vi "ProEM.vi"() -> ()   [LabVIEW 2012]
uses:
  <vilib>/Utility/error.llb/DialogType.ctl
  <vilib>/Platform/TimedLoop/XDataNode/timing_clust.ctl
  <vilib>/Platform/TimedLoop/XDataNode/nitl_modes.ctl
  <vilib>/Platform/TimedLoop/XDataNode/wakeup.ctl
  SITK/Documents/SIToolkit/LabVIEW/Examples2012_4_1_0_4/Open-Close/CamHandle.vi
  <vilib>/platform/TimedLoop/XDataNode/XDataNode.xnode
  <vilib>/Platform/TimedLoop/XDataNode/XDNodeRunTimeDep.lvlib
panel:
  in  "Tab Control":enum32{"Control", "Advanced"}(tab)
  in  "?":u16(ring) items=["Debug", "Bulb Trigger", "Free Run"]
  out "Image Monitor":u16[][](graph)
  in  "Number of Accumulations":u32=1
  in  "Number of Images":u32=1
  in  "Time Between Shots":dbl
  in  "Acquire / Focus Flag":u32(ring)=2 items=["Synchronous Focus Mode"=1, "Synchronous NFrame Mode"=2, "Asynchronous Mode"=3, "Sequence Mode"=4]
  in  "Errors":errorcluster
  in  "ADC Gain":i32=-1 min=-1 step=1
  in  "ADC Speed":i32=-1 min=-3 step=1
  in  "Exposure (sec)":dbl format="%.3f"
  in  "Timing Mode":u32(ring)=4 items=["Free Run"=1, "Trigger First"=2, "Strobe"=3, "Bulb"=4, "Variable"=5, "Flash"=6]
  in  "Trigger Edge":u32(ring)=1 items=["Rising"=1, "Falling"=2]
  in  "stop":bool
  in  "Camera Handle 2":u32
  in  "File and Display Name 2":string
  in  "error in (no error) 2":errorcluster
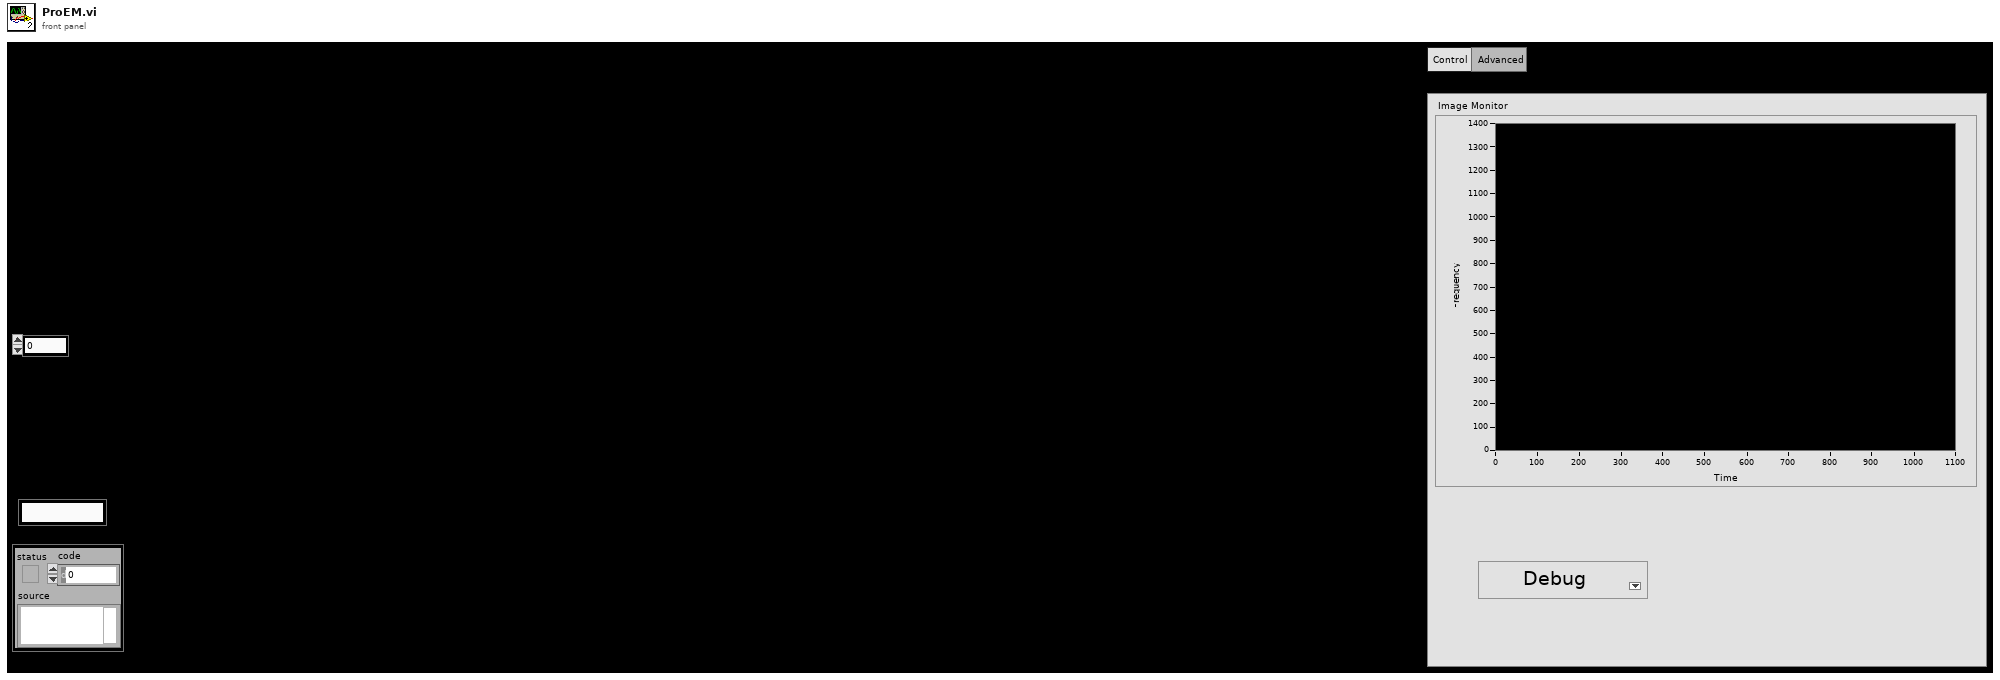
[diagram p1: front panel]
types:
  T1 = typedef "XDNodeRunTimeDep.lvlib/timing_clust.ctl" = cluster{"Expected End [f-1]":u64, "Actual End [f-1]":u64, "Finished Late? [f-1]":bool, "Expected End [i-1]":u64, "Actual End [i-1]":u64, "Finished Late? [i-1]":bool, "Expected Start [i]":u64, "Actual Start [i]":u64, "Expected Start [f]":u64, "Actual Start [f]":u64, "Source Name":string, "Structure Name":string, "Period":i64, "Deadline":i64, "Offset":i64, "Start":i64, "Priority":i32, "Timeout":i32, "Mode":T2, "Wakeup Reason":T3, "Error":errorcluster, "Source Type":string, "Secondary Source Type":string, "Global End Time":u64, "Global Start Time":u64, "Frame Duration":u64, "Iteration Duration":u64, "Assigned CPU":i32, "I/O Scan Engine Mode":u32}
  T2 = typedef "XDNodeRunTimeDep.lvlib/nitl_modes.ctl" = enum32{"No Change", "Process missed periods, maintain original phase", "Discard missed periods, maintain original phase", "Process missed periods, ignore original phase", "Discard missed periods, ignore original phase"}
  T3 = typedef "XDNodeRunTimeDep.lvlib/wakeup.ctl" = enum32{"Normal", "Aborted", "Asynchronous wakeup", "Timing source error", "Timed loop error", "Timeout"}
  T4 = typedef "DialogType.ctl" = u16
  T5 = cluster{"Camera Handle":u32, "File Handle":u32, "Display Handle":u32, "Image Handle":u32}
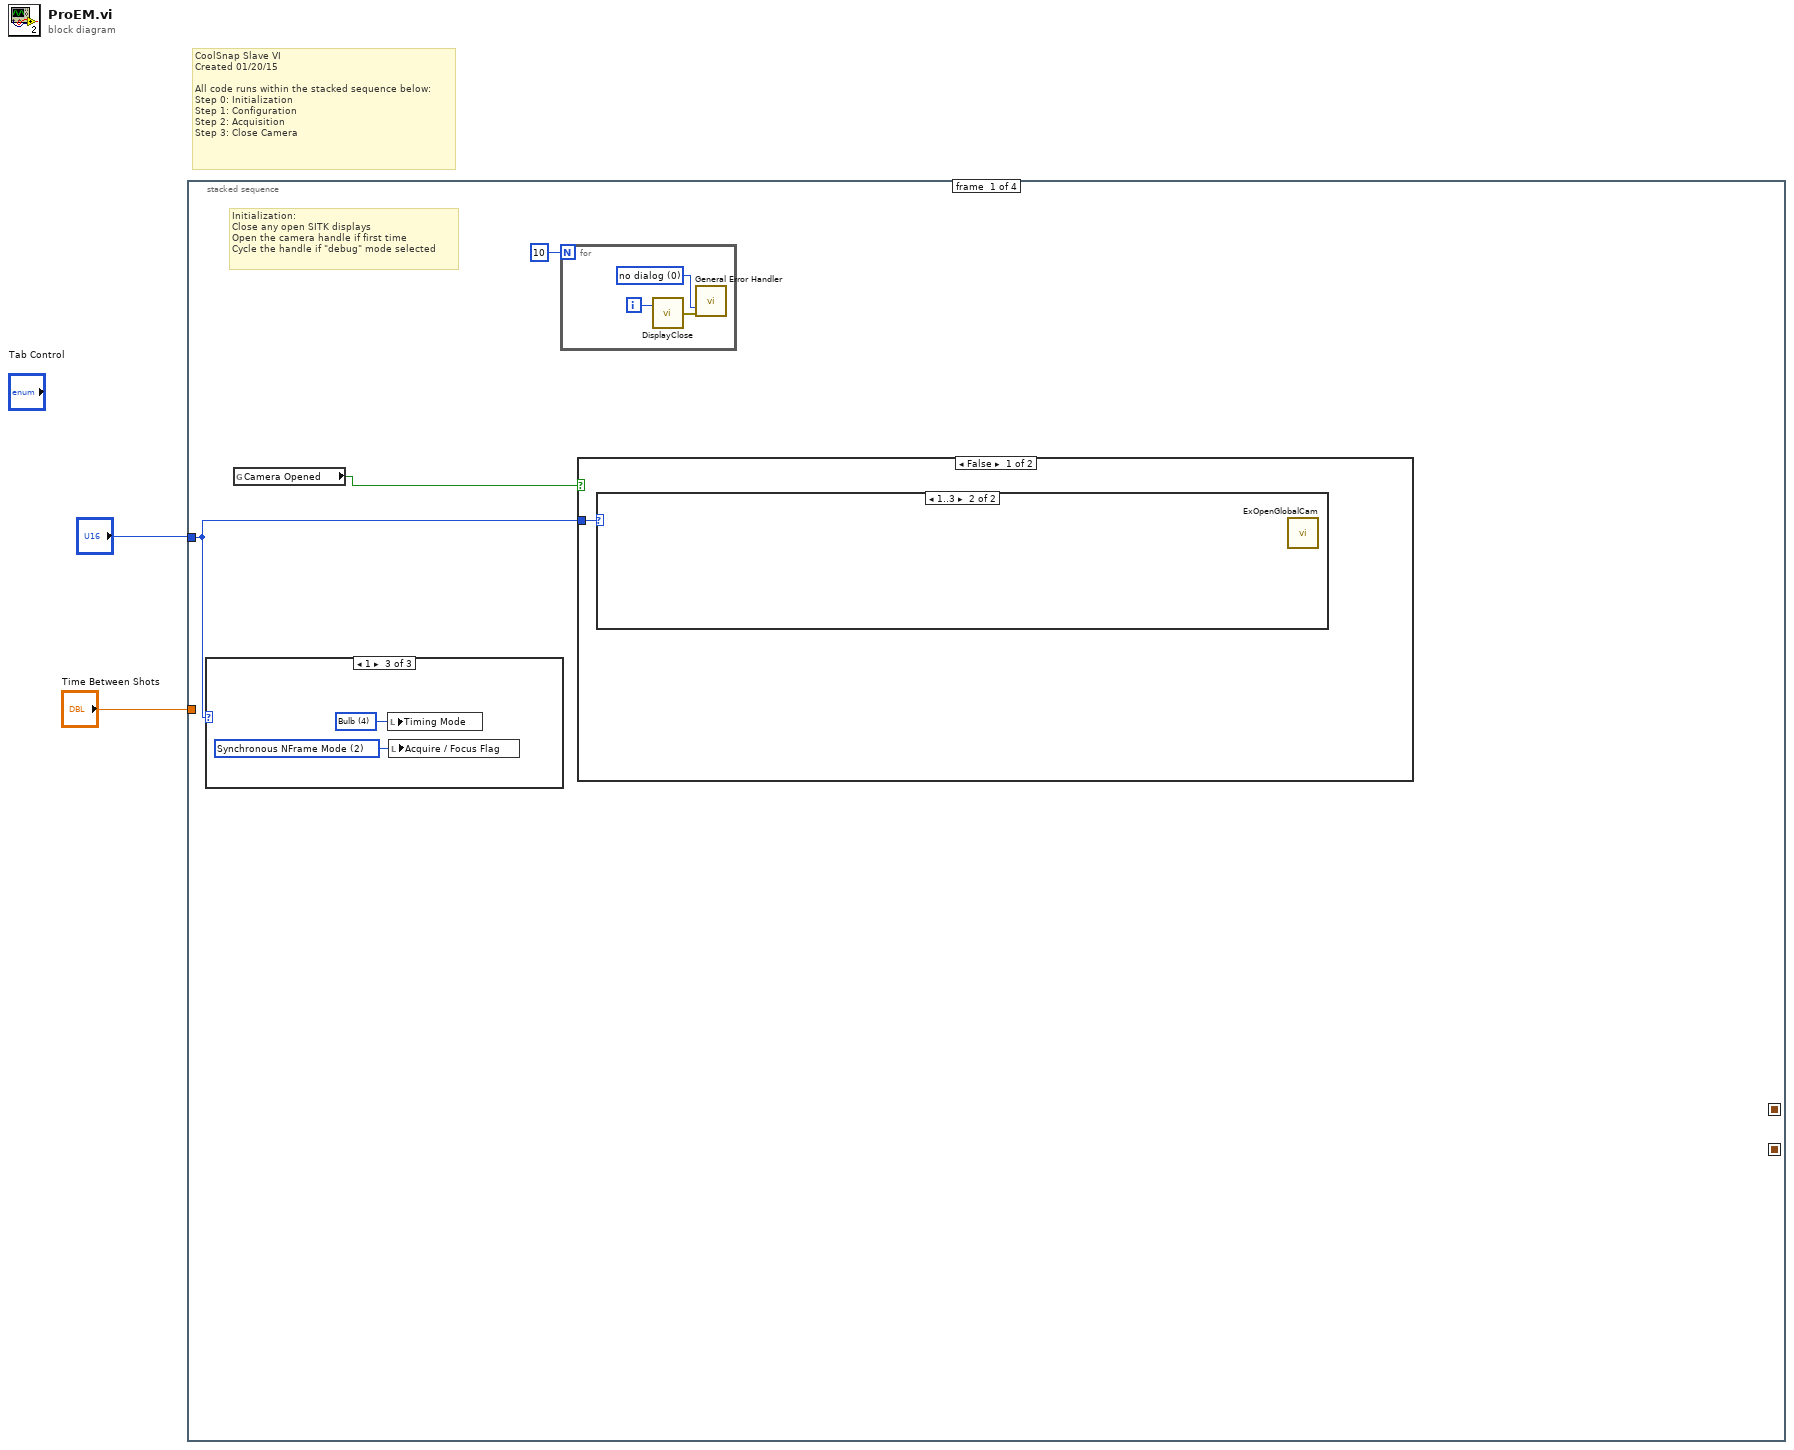
[diagram p0: block diagram]
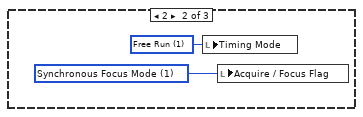
[diagram p3: hidden frame]
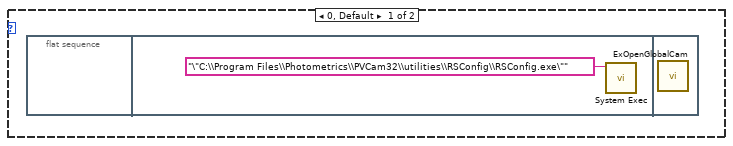
[diagram p4: hidden frame]
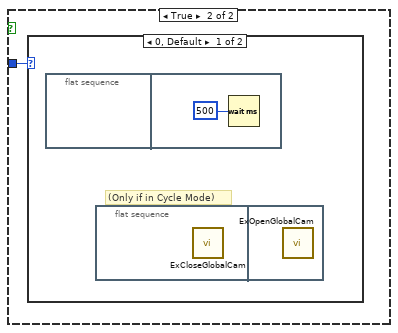
[diagram p5: hidden frame]
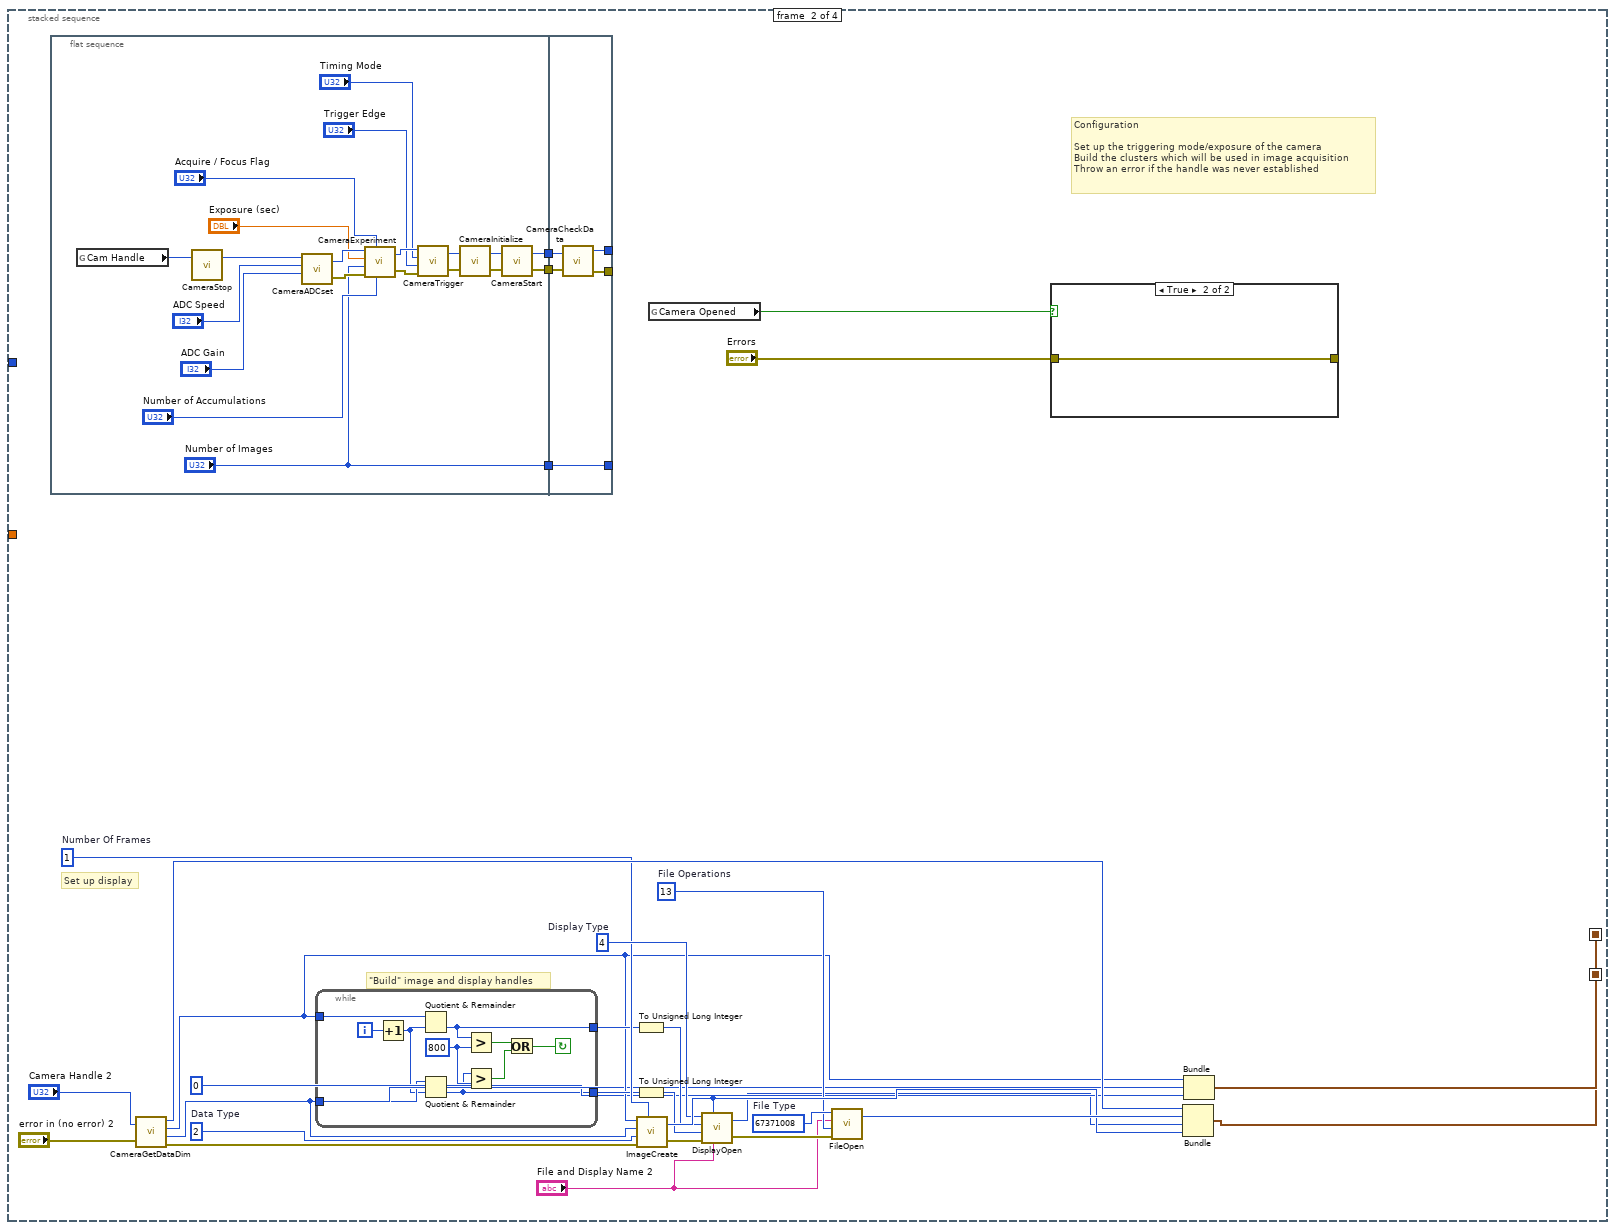
[diagram p7: hidden frame]
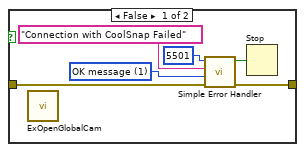
[diagram p8: hidden frame]
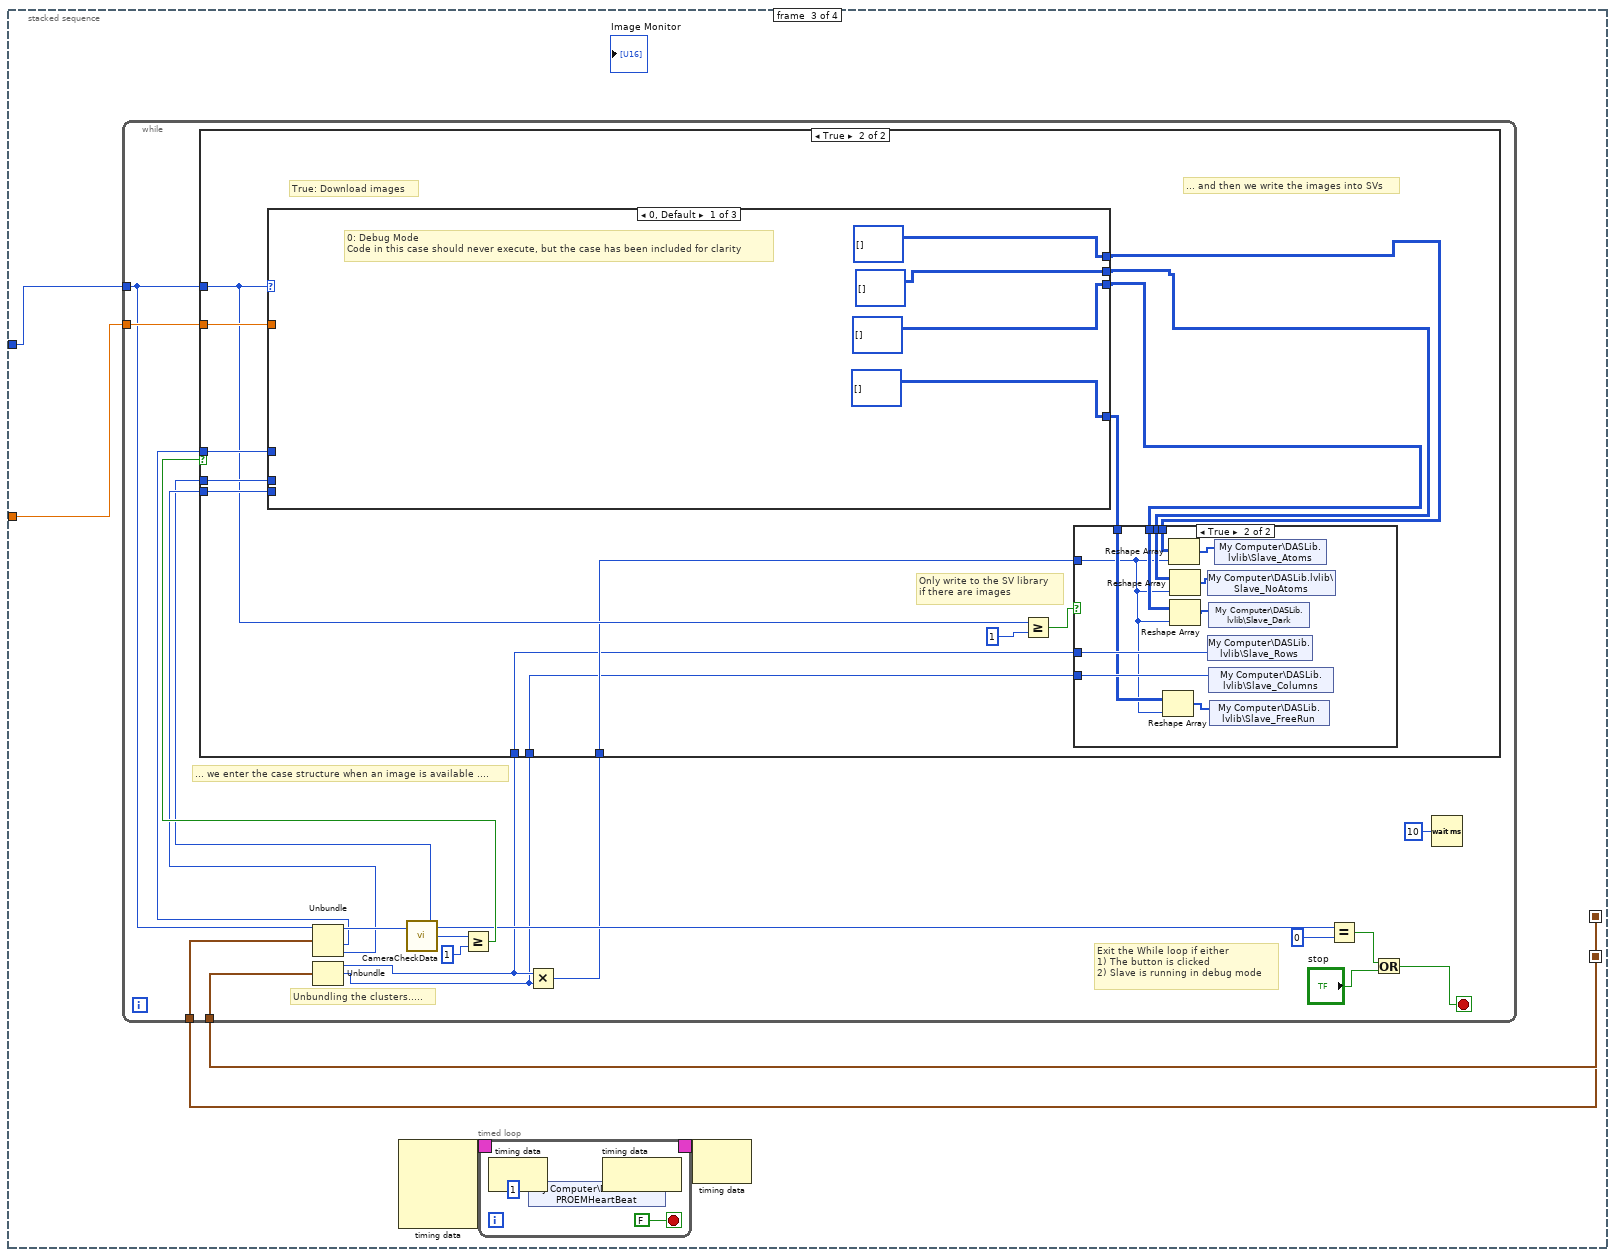
[diagram p9: hidden frame]
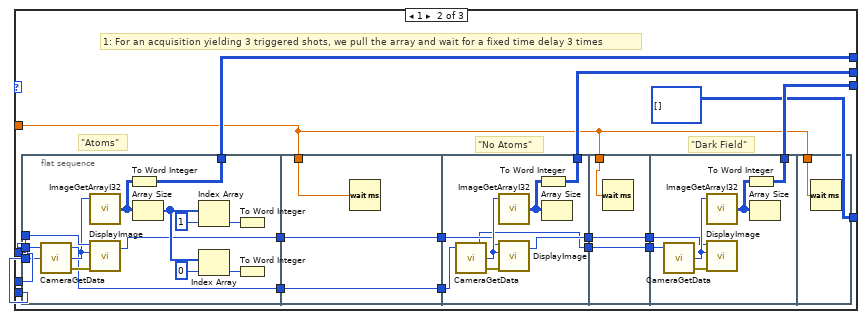
[diagram p12: hidden frame]
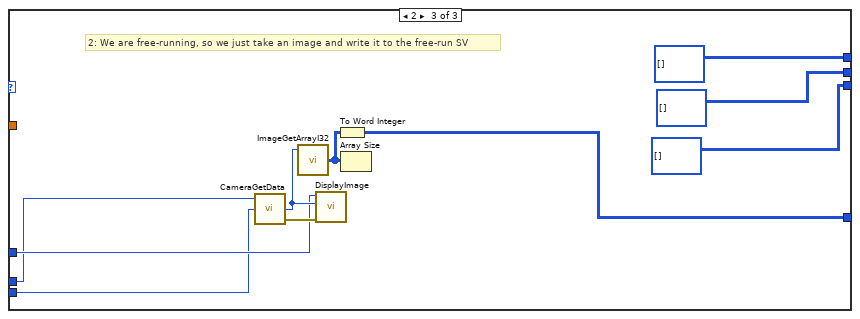
[diagram p13: hidden frame]
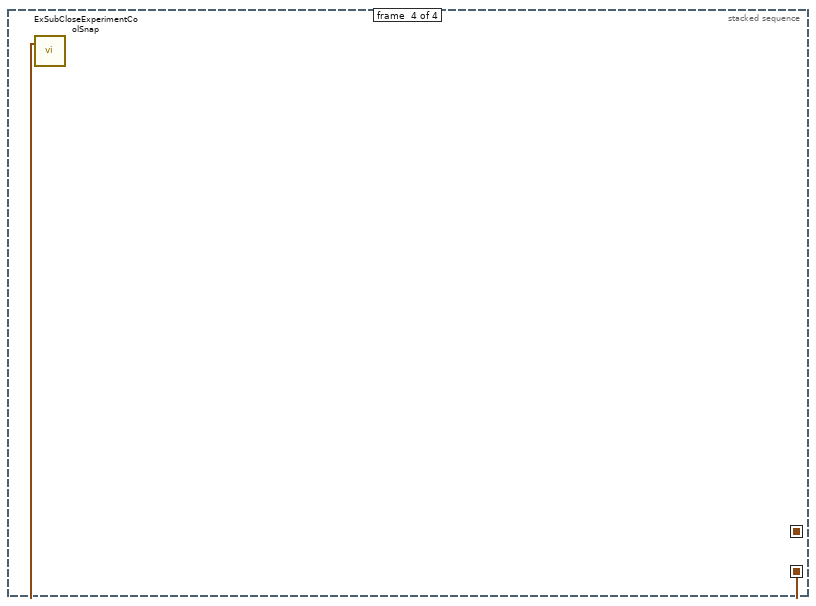
[diagram p14: hidden frame]
diagram:
  # "CoolSnap Slave VI\nCreated 01/20/15\n\nAll code runs within the stacked sequence below:\nStep 0: Initialization\nStep 1: Configuration\nStep 2: Acquisition\nStep 3: Close Camera"
  n1 = stacked-sequence {
    seq-local: [_ w20 _ _] -> [_ _ w93 _]
    seq-local: [_ w19 _ _] -> [_ _ w90 w209]
    tunnel: "?" -> [w3 _ w92 _]
    tunnel: "Time Between Shots" -> [_ _ w91 _]
    frame #0 {
      # "Initialization:\nClose any open SITK displays\nOpen the camera handle if first time\nCycle the handle if \"debug\" mode selected"
      n2 = case shown="1" w3 {
        frame 0, Default {
        }
        frame 2 {
          w6 = u32 1 items=["Synchronous Focus Mode"=1, "Synchronous NFrame Mode"=2, "Asynchronous Mode"=3, "Sequence Mode"=4] ("Acquire / Focus Flag")
          w7 = u32 1 items=["Free Run"=1, "Trigger First"=2, "Strobe"=3, "Bulb"=4, "Variable"=5, "Flash"=6] ("Timing Mode")
          n3 = local write "Timing Mode"(w7) -> ()
          n4 = local write "Acquire / Focus Flag"(w6) -> ()
        }
        frame 1 {
          w8 = u32 2 items=["Synchronous Focus Mode"=1, "Synchronous NFrame Mode"=2, "Asynchronous Mode"=3, "Sequence Mode"=4] ("Acquire / Focus Flag")
          w9 = u32 4 items=["Free Run"=1, "Trigger First"=2, "Strobe"=3, "Bulb"=4, "Variable"=5, "Flash"=6] ("Timing Mode")
          n5 = local write "Timing Mode"(w9) -> ()
          n6 = local write "Acquire / Focus Flag"(w8) -> ()
        }
      }
      n7 = global read "CamHandle.vi" "Camera Opened"() -> (w4:bool)
      n8 = for {
        N: 10 -> [_]
        i -> [w16]
        w14 = T4 0 items=["no dialog", "OK message", "continue or stop message", "OK message + warnings", "continue/stop + warnings"] ("type of dialog (OK msg:1)")
        n9 = call <userlib>:"DisplayClose.vi"("Display Handle"=w16) -> ("error out"=w15:errorcluster)  [unwired: 1 in]
        n10 = call <vilib>:"General Error Handler.vi"("type of dialog (OK msg:1)"=w14, "error in (no error)"=w15) -> ()  [unwired: 9 in, 5 out]
      }
      n11 = case shown="False" w4 {
        tunnel: w3 -> [w10 w12]
        frame False {
          n12 = case shown="1..3" w10 {
            frame 0, Default {
              n13 = flat-sequence {
                frame #0 {
                }
                frame #1 {
                  n14 = call <vilib>:"System Exec.vi"("command line"="\"C:\\Program Files\\Photometrics\\PVCam32\\utilities\\RSConfig\\RSConfig.exe\"") -> ()  [unwired: 7 in, 4 out]
                }
                frame #2 {
                  n15 = call "ExOpenGlobalCam.vi"() -> ()  [unwired: 1 in]
                }
              }
            }
            frame 1..3 {
              n16 = call "ExOpenGlobalCam.vi"() -> ()  [unwired: 1 in]
            }
          }
        }
        frame True {
          n17 = case shown="0, Default" w12 {
            frame 0, Default {
              # "(Only if in Cycle Mode)"
              n18 = flat-sequence {
                frame #0 {
                }
                frame #1 {
                  n19 = Wait (ms)(milliseconds to wait=u32 500) -> ()  [unwired: 1 out]
                }
              }
              n20 = flat-sequence {
                frame #0 {
                  n21 = call "ExCloseGlobalCam.vi"() -> ()  [unwired: 1 in]
                }
                frame #1 {
                  n22 = call "ExOpenGlobalCam.vi"() -> ()  [unwired: 1 in]
                }
              }
            }
            frame 1..3 {
            }
          }
        }
      }
    }
    frame #1 {
      w29 = u32 1  # Number Of Frames
      w30 = u32 4  # Display Type
      w31 = u32 2  # Data Type
      w33 = 13  # File Operations
      w34 = 67371008  # File Type
      # "Configuration\n\nSet up the triggering mode/exposure of the camera\nBuild the clusters which will be used in image acquisition\nThrow an error if the handle was never established"
      # "\"Build\" image and display handles"
      # "Set up display"
      n23 = flat-sequence {
        tunnel: ["Number of Images"] -> w45
        tunnel: [w70] -> w44
        tunnel: [w69] -> w43
        tunnel: [w83] -> _
        tunnel: [w87] -> _
        tunnel: w45 -> [w87]
        tunnel: w44 -> [w86]
        tunnel: w43 -> [w85]
        tunnel: [w84] -> _
        frame #0 {
          n24 = global read "CamHandle.vi" "Cam Handle"() -> (w64:u32)
          n25 = call <userlib>:"CameraStop.vi"("Camera Handle"=w64) -> ("Camera Handle"=w65:u32)  [unwired: 1 in, 1 out]
          n26 = call <userlib>:"CameraADCset.vi"("ADC Gain"="ADC Gain", "ADC Speed"="ADC Speed", "Camera Handle"=w65) -> ("error out"=w80:errorcluster, "Camera Handle"=w82:u32)  [unwired: 3 in]
          n27 = call <userlib>:"CameraExperiment.vi"("Number of Accumulations"="Number of Accumulations", "Acquire / Focus Flag"="Acquire / Focus Flag", "error in"=w80, "Number of Images"="Number of Images", "Exposure (sec)"="Exposure (sec)", "Camera Handle"=w82) -> ("error out"=w74:errorcluster, "Camera Handle"=w75:u32)
          n28 = call <userlib>:"CameraTrigger.vi"("error in"=w74, "Trigger Edge"="Trigger Edge", "Timing Mode"="Timing Mode", "Camera Handle"=w75) -> ("error out"=w66:errorcluster, "Camera Handle"=w71:u32)
          n29 = call <userlib>:"CameraInitialize.vi"("error in"=w66, "Camera Handle"=w71) -> ("error out"=w68:errorcluster, "Camera Handle"=w67:u32)
          n30 = call <userlib>:"CameraStart.vi"("error in"=w68, "Camera Handle"=w67) -> ("error out"=w69:errorcluster, "Camera Handle"=w70:u32)
        }
        frame #1 {
          n31 = call <userlib>:"CameraCheckData.vi"("Camera Handle"=w86, "error in"=w85) -> ("Camera Handle"=w83:u32, "error out"=w84:errorcluster)  [unwired: 1 out]
        }
      }
      n32 = call <userlib>:"CameraGetDataDim.vi"("Camera Handle"="Camera Handle 2", "error in"="error in (no error) 2") -> ("Camera Handle"=w37:u32, "Xdim"=w24:u32, "Ydim"=w23:u32, "error out"=w42:errorcluster)
      n33 = while {
        tunnel: w24 -> [w61]
        tunnel: w23 -> [w60]
        tunnel: [w55] -> w28
        tunnel: [w54] -> w27
        i -> [w59]
        stop <- w56 continue-if-true
        w62 = 800
        n34 = Increment(x=w59) -> (x+1=w53:i32)
        n35 = Quotient & Remainder(x=w61, y=w53) -> (floor(x/y)=w55:u32)  [unwired: 1 out]
        n36 = Quotient & Remainder(x=w60, y=w53) -> (floor(x/y)=w54:u32)  [unwired: 1 out]
        n37 = Greater?(x=w55, y=w62) -> (0:w58:bool)
        n38 = Greater?(x=w54, y=w62) -> (0:w57:bool)
        n39 = Or(x=w58, y=w57) -> (x .or. y?=w56:bool)
      }
      n40 = To Unsigned Long Integer(number=w28) -> (unsigned 32bit integer=w26:u32)
      n41 = To Unsigned Long Integer(number=w27) -> (unsigned 32bit integer=w25:u32)
      n42 = call <userlib>:"ImageCreate.vi"("X dimension"=w24, "Y dimension"=w23, "Data Type"=w31, "error in"=w42, "Number Of Frames"=w29) -> ("Image Handle"=w35:u32, "error out"=w41:errorcluster)
      n43 = global read "CamHandle.vi" "Camera Opened"() -> (w18:bool)
      n44 = call <userlib>:"DisplayOpen.vi"("Display Title"="File and Display Name 2", "Image Handle"=w35, "error in"=w41, "Display Height"=w25, "Display Width"=w26, "Display Type"=w30) -> ("error out"=w40:errorcluster, "Display Handle"=w21:u32)
      n45 = call <userlib>:"FileOpen.vi"("error in"=w40, "File Operations"=w33, "FileName"="File and Display Name 2", "File Type"=w34) -> ("File Handle"=w36:u32)  [unwired: 1 out]
      n46 = case shown="True" w18 {
        tunnel: [w50 w52] -> _
        tunnel: "Errors" -> [w46 w52]
        frame False {
          w51 = u16 1 items=["no dialog", "OK message", "continue or stop message"] ("type of dialog (OK msg:1)")
          n47 = call "ExOpenGlobalCam.vi"() -> ()  [unwired: 1 in]
          n48 = call <vilib>:"Simple Error Handler.vi"("error code (no error:0)"=5501, "error source (\" \")"="Connection with CoolSnap Failed", "type of dialog (OK msg:1)"=w51, "error in (no error)"=w46) -> ("error?"=w48:bool, "error out"=w50:errorcluster)  [unwired: 1 in, 3 out]
          n49 = Stop(stop? (T)=w48) -> ()
        }
        frame True {
        }
      }
      n50 = Bundle("Camera Handle"=w37, "File Handle"=w36, "Display Handle"=w21, "Image Handle"=w35) -> (w19:T5)  [unwired: 1 in]
      n51 = Bundle("Xdim"=w24, "Ydim"=w23, 0) -> (w20:cluster{"Xdim":u32, "Ydim":u32, i32})  [unwired: 1 in]
    }
    frame #2 {
      n52 = while {
        tunnel: w93 -> [w118]
        tunnel: w90 -> [w117]
        tunnel: w92 -> [w104]
        tunnel: w91 -> [w105]
        stop <- w107 stop-if-true
        # "... we enter the case structure when an image is available ...."
        # "Unbundling the clusters....."
        # "Exit the While loop if either\n1) The button is clicked\n2) Slave is running in debug mode"
        n53 = Unbundle(w117) -> ("Camera Handle"=w116:u32, "Display Handle"=w111:u32, "Image Handle"=w112:u32)  [unwired: 1 out]
        n54 = Unbundle(w118) -> ("Xdim"=w102:u32, "Ydim"=w101:u32)  [unwired: 1 out]
        n55 = call <userlib>:"CameraCheckData.vi"("Camera Handle"=w116) -> ("Camera Handle"=w110:u32, "Number Of Frames Available"=w115:i32)  [unwired: 1 in, 1 out]
        n56 = Greater Or Equal?(x=w115, y=1) -> (x >= y?=w113:bool)
        n57 = Multiply(x=w102, y=w101) -> (x*y=w103:u32)
        n58 = case shown="True" w113 {
          tunnel: w110 -> [_ w131]
          tunnel: w112 -> [_ w130]
          tunnel: w111 -> [_ w132]
          tunnel: w104 -> [_ w126]
          tunnel: w105 -> [_ w129]
          tunnel: w103 -> [_ w125]
          tunnel: w102 -> [_ w124]
          tunnel: w101 -> [_ w123]
          frame False {
            # "False: Keep waiting for images"
          }
          frame True {
            # "Only write to the SV library \nif there are images"
            # "... and then we write the images into SVs"
            # "True: Download images"
            n59 = case shown="0, Default" w126 {
              tunnel: w132 -> [_ w163 w205]
              tunnel: w131 -> [_ w162 w204]
              tunnel: w130 -> [_ w161 w203]
              tunnel: w129 -> [_ w149 _]
              tunnel: [i16[][] [] w152 i16[][] []] -> w122
              tunnel: [i16[][] [] w151 i16[][] []] -> w121
              tunnel: [i16[][] [] w150 i16[][] []] -> w120
              tunnel: [i16[][] [] i16[][] [] w199] -> w119
              frame 0, Default {
                # "0: Debug Mode\nCode in this case should never execute, but the case has been included for clarity"
              }
              frame 1 {
                # "\"Dark Field\""
                # "\"No Atoms\""
                # "\"Atoms\""
                # "1: For an acquisition yielding 3 triggered shots, we pull the array and wait for a fixed time delay 3 times"
                n60 = flat-sequence {
                  tunnel: w163 -> [w177]
                  tunnel: w162 -> [w176]
                  tunnel: w161 -> [w175]
                  tunnel: [w166] -> w159
                  tunnel: [w165] -> w154
                  tunnel: [w164] -> w152
                  tunnel: w149 -> [w180]
                  tunnel: [w179] -> w160
                  tunnel: w159 -> [w179]
                  tunnel: w154 -> [w178]
                  tunnel: [w178] -> w153
                  tunnel: w160 -> [w185]
                  tunnel: [w184] -> w157
                  tunnel: [w183] -> w156
                  tunnel: w153 -> [w182]
                  tunnel: [w181] -> w151
                  tunnel: [w191] -> w158
                  tunnel: w157 -> [w191]
                  tunnel: w156 -> [w190]
                  tunnel: [w190] -> w155
                  tunnel: w149 -> [w189]
                  tunnel: w158 -> [w194]
                  tunnel: w155 -> [w193]
                  tunnel: [w192] -> w150
                  tunnel: w149 -> [w198]
                  frame #0 {
                    n61 = call <userlib>:"CameraGetData.vi"("Data Handle"=w175, "Camera Handle"=w176) -> ("error out"=w174:errorcluster, "Data Handle"=w173:u32, "Camera Handle"=w165:u32)  [unwired: 1 in]
                    n62 = call <userlib>:"ImageGetArrayI32.vi"("Image Handle"=w173) -> ("Array int 32"=w167:i32[][])  [unwired: 2 in, 2 out]
                    n63 = call <userlib>:"DisplayImage.vi"("error in"=w174, "Image Handle"=w173, "Display Handle"=w177) -> ("Display Handle"=w166:u32)  [unwired: 1 in, 1 out]
                    n64 = To Word Integer(number=w167) -> (16bit integer=w164:i16[][])
                    n65 = Array Size(array=w167) -> (size(s)=w168:i32[])
                    n66 = Index Array(array=w168, index=1) -> (element=w169:i32)
                    n67 = Index Array(array=w168, index=0) -> (element=w170:i32)
                    n68 = To Word Integer(number=w169) -> ()  [unwired: 1 out]
                    n69 = To Word Integer(number=w170) -> ()  [unwired: 1 out]
                  }
                  frame #1 {
                    n70 = Wait (ms)(milliseconds to wait=w180) -> ()  [unwired: 1 out]
                  }
                  frame #2 {
                    n71 = call <userlib>:"CameraGetData.vi"("Camera Handle"=w182) -> ("error out"=w188:errorcluster, "Data Handle"=w187:u32, "Camera Handle"=w183:u32)  [unwired: 2 in]
                    n72 = call <userlib>:"ImageGetArrayI32.vi"("Image Handle"=w187) -> ("Array int 32"=w186:i32[][])  [unwired: 2 in, 2 out]
                    n73 = call <userlib>:"DisplayImage.vi"("error in"=w188, "Image Handle"=w187, "Display Handle"=w185) -> ("Display Handle"=w184:u32)  [unwired: 1 in, 1 out]
                    n74 = To Word Integer(number=w186) -> (16bit integer=w181:i16[][])
                    n75 = Array Size(array=w186) -> ()  [unwired: 1 out]
                  }
                  frame #3 {
                    n76 = Wait (ms)(milliseconds to wait=w189) -> ()  [unwired: 1 out]
                  }
                  frame #4 {
                    n77 = call <userlib>:"CameraGetData.vi"("Camera Handle"=w193) -> ("error out"=w197:errorcluster, "Data Handle"=w196:u32)  [unwired: 2 in, 1 out]
                    n78 = call <userlib>:"ImageGetArrayI32.vi"("Image Handle"=w196) -> ("Array int 32"=w195:i32[][])  [unwired: 2 in, 2 out]
                    n79 = call <userlib>:"DisplayImage.vi"("error in"=w197, "Image Handle"=w196, "Display Handle"=w194) -> ()  [unwired: 1 in, 2 out]
                    n80 = To Word Integer(number=w195) -> (16bit integer=w192:i16[][])
                    n81 = Array Size(array=w195) -> ()  [unwired: 1 out]
                  }
                  frame #5 {
                    n82 = Wait (ms)(milliseconds to wait=w198) -> ()  [unwired: 1 out]
                  }
                }
              }
              frame 2 {
                # "2: We are free-running, so we just take an image and write it to the free-run SV"
                n83 = call <userlib>:"CameraGetData.vi"("Data Handle"=w203, "Camera Handle"=w204) -> ("error out"=w208:errorcluster, "Data Handle"=w207:u32)  [unwired: 1 in, 1 out]
                n84 = call <userlib>:"ImageGetArrayI32.vi"("Image Handle"=w207) -> ("Array int 32"=w206:i32[][])  [unwired: 2 in, 2 out]
                n85 = call <userlib>:"DisplayImage.vi"("error in"=w208, "Image Handle"=w207, "Display Handle"=w205) -> ()  [unwired: 1 in, 2 out]
                n86 = To Word Integer(number=w206) -> (16bit integer=w199:i16[][])
                n87 = Array Size(array=w206) -> ()  [unwired: 1 out]
              }
            }
            n88 = Greater Or Equal?(x=w126, y=1 ("index")) -> (x >= y?=w127:bool)
            n89 = case shown="True" w127 {
              tunnel: w121 -> [_ w143]
              tunnel: w122 -> [_ w142]
              tunnel: w120 -> [_ w141]
              tunnel: w125 -> [_ w133]
              tunnel: w124 -> [_ w137]
              tunnel: w123 -> [_ w136]
              tunnel: w119 -> [_ w134]
              frame False {
                # "No bombarding the SV library with free-run\nimages!"
              }
              frame True {
                n90 = Reshape Array(w134, w133) -> (w135:i16[])
                n91 = Reshape Array(w142, w133) -> (w140:i16[])
                n92 = Reshape Array(w143, w133) -> (w139:i16[])
                n93 = Reshape Array(w141, w133) -> (w138:i16[])
                n94 = shared-variable "My Computer\\DASLib.lvlib\\Slave_NoAtoms"(w139) -> ()  [unwired: 1 in, 1 out]
                n95 = shared-variable "My Computer\\DASLib.lvlib\\Slave_Rows"(w137) -> ()  [unwired: 1 in, 1 out]
                n96 = shared-variable "My Computer\\DASLib.lvlib\\Slave_Dark"(w138) -> ()  [unwired: 1 in, 1 out]
                n97 = shared-variable "My Computer\\DASLib.lvlib\\Slave_Columns"(w136) -> ()  [unwired: 1 in, 1 out]
                n98 = shared-variable "My Computer\\DASLib.lvlib\\Slave_FreeRun"(w135) -> ()  [unwired: 1 in, 1 out]
                n99 = shared-variable "My Computer\\DASLib.lvlib\\Slave_Atoms"(w140) -> ()  [unwired: 1 in, 1 out]
              }
            }
          }
        }
        n100 = Equal?(x=w104, y=0 ("index")) -> (x = y?=w108:bool)
        n101 = Or(x=w108, y="stop") -> (x .or. y?=w107:bool)
        n102 = Wait (ms)(milliseconds to wait=u32 10) -> ()  [unwired: 1 out]
      }
      n103 = node-c288() -> (w89:T1)  [unwired: 4 in]
      n104 = timed-loop {
        timing: w89 -> [_]
        timing-out: [_] -> w88
        stop <- FALSE stop-if-true
        n105 = node-c288() -> ()  [unwired: 1 in, 1 out]
        n106 = shared-variable "My Computer\\DASLib.lvlib\\PROEMHeartBeat"(i16 1 ("PFHeartBeat")) -> ()  [unwired: 1 in, 1 out]
        n107 = node-c288() -> ()  [unwired: 1 in, 1 out]
      }
      n108 = node-c288(w88) -> ()  [unwired: 1 out]
    }
    frame #3 {
      n109 = call "ExSubCloseExperimentCoolSnap.vi"("Handles In"=w209) -> ()  [unwired: 1 in, 1 out]
    }
  }
